vi "Axes_n_Buttons_Global.vi"() -> ()   [LabVIEW 2019]
panel:
  out "AutoRight":dbl
  out "AutoLeft":dbl
  out "DrButton5":bool
  out "DrButton4":bool
  out "DrButton2":bool
  out "DrButton0":bool
  out "DrAxis4":dbl
  out "DrAxis3":dbl
  out "DrAxis2":dbl
  out "DrAxis1":dbl
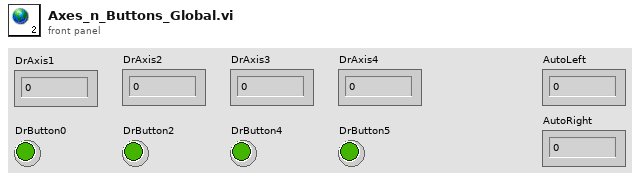
[diagram p1: front panel]
diagram:
